vi "Initilize RxTx Array.vi"(8 "error in (no error)":errorcluster, 11 "SPARC4_AC in":refnum<class "S4ACS_GUI.lvclass">) -> (0 "error out":errorcluster, 3 "SPARC4_AC out":refnum<class "S4ACS_GUI.lvclass">)   [LabVIEW 2012, in "S4ACS_GUI.lvclass"]
uses:
  S4ACS_GUI.lvclass
  RxTx/RxTx.lvclass
panel:
  in  "RxTx.lvclass":refnum<class "RxTx.lvclass">=refnum
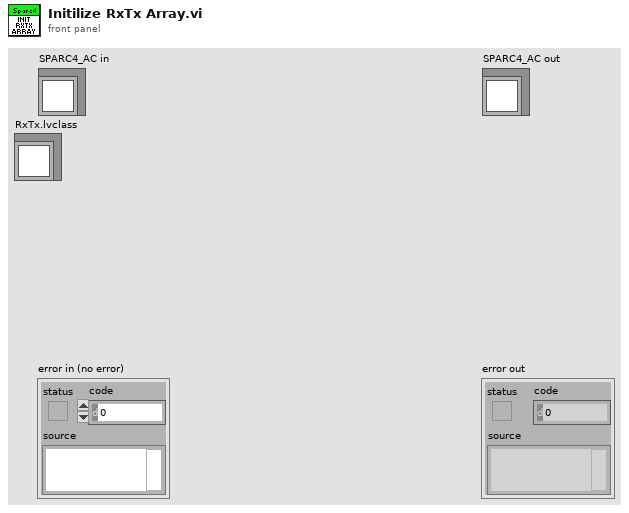
[diagram p1: front panel]
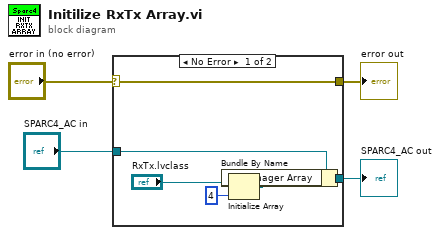
[diagram p0: block diagram]
diagram:
  n1 = case shown="No Error" "error in (no error)" {
    selector: "error in (no error)" -> [w10 w12]
    tunnel: [w10 w12] -> w3
    tunnel: [w7 w11] -> w1
    tunnel: "SPARC4_AC in" -> [w6 w11]
    frame No Error {
      n2 = Initialize Array("RxTx.lvclass", 4 ("dimension size")) -> (w5:refnum<class "RxTx.lvclass">[])
      n3 = Bundle By Name(cluster=w6, "ChManager Array"=w5) -> (w7:refnum<class "S4ACS_GUI.lvclass">)
    }
    frame Error {
    }
  }
  "error out" <- w3
  "SPARC4_AC out" <- w1
